vi "User log event LV2.vi"(0 "User Data":string[][](array[string]), 11 "Error in":errorcluster, 13 "Operation":T1) -> (4 "User data ref":refnum<user-event>, 15 "Error out":errorcluster)   [LabVIEW 2020, in "PSRR Monitor.lvlib"]
doc: "This LV2 is used as a user event which is used transmit the error data to the error table VI from the main producer consumer vi"
uses:
  PSRR Monitor.lvlib
  Typedefs/User LV2 operations.ctl
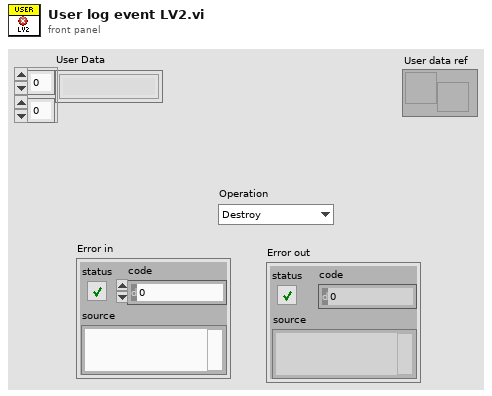
[diagram p1: front panel]
types:
  T1 = typedef "PSRR Monitor.lvlib/User LV2 operations.ctl" = enum16{"Destroy", "Get ref", "Generate", "Create"}
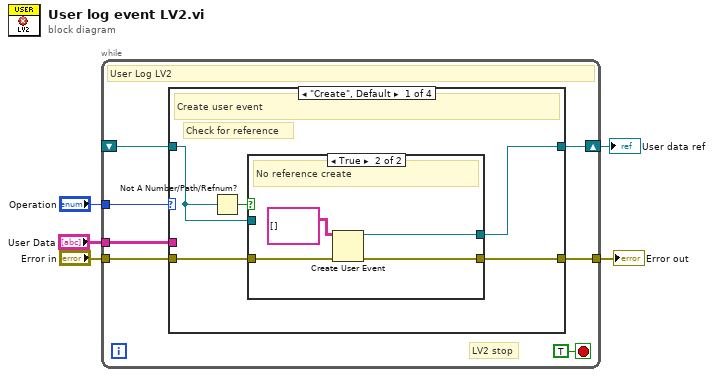
[diagram p0: block diagram]
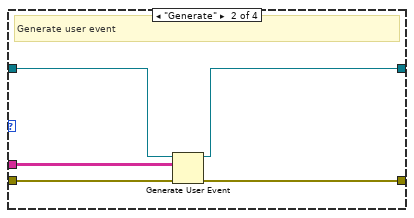
[diagram p3: hidden frame]
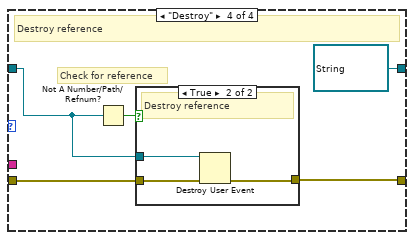
[diagram p5: hidden frame]
diagram:
  n1 = while {
    tunnel: "Operation" -> [w11]
    tunnel: "Error in" -> [w10]
    tunnel: [w9] -> w3
    tunnel: "User Data" -> [w8]
    shift-right: [w7] -> w1
    shift-left: _ -> [w6]
    stop <- TRUE stop-if-true
    # "LV2 stop"
    # "User Log LV2"
    n2 = case shown="\"Create\", Default" w11 {
      tunnel: w10 -> [w17 w28 w30 w34]
      tunnel: [w16 w27 w30 w33] -> w9
      tunnel: w8 -> [_ w24 _ _]
      tunnel: [w15 w25 w29 refnum<user-event> refnum ("User Data")] -> w7
      tunnel: w6 -> [w13 w26 w29 w32]
      frame "Create", Default {
        # "Check for reference"
        # "Create user event"
        n3 = Not A Number/Path/Refnum?(number/path/refnum=w13) -> (NaN/Path/Refnum?=w14:bool)
        n4 = case shown="True" w14 {
          tunnel: w17 -> [w18 w23]
          tunnel: [w18 w22] -> w16
          tunnel: [w19 w21] -> w15
          tunnel: w13 -> [w19 _]
          frame False {
            # "Continue"
          }
          frame True {
            # "No reference create"
            n5 = Create User Event(user event datatype=string[][] [] ("User Data"), error in=w23) -> (user event=w21:refnum<user-event>, error out=w22:errorcluster)
          }
        }
      }
      frame "Generate" {
        # "Generate user event"
        n6 = Generate User Event(user event=w26, event data cluster=w24, error in=w28) -> (user event out=w25:refnum<user-event>, error out=w27:errorcluster)  [unwired: 1 in]
      }
      frame "Get ref" {
        # "Get user event reference"
      }
      frame "Destroy" {
        # "Check for reference"
        # "Destroy reference"
        n7 = Not A Number/Path/Refnum?(number/path/refnum=w32) -> (NaN/Path/Refnum?=w35:bool)
        n8 = case shown="True" w35 {
          tunnel: w34 -> [w36 w39]
          tunnel: [w36 w38] -> w33
          tunnel: w32 -> [_ w37]
          frame False {
          }
          frame True {
            # "Destroy reference"
            n9 = Destroy User Event(user event=w37, error in=w39) -> (error out=w38:errorcluster)
          }
        }
      }
    }
  }
  "Error out" <- w3
  "User data ref" <- w1
